vi "secuenciabloqueante.vi"() -> ()   [LabVIEW 2020]
panel:
  out "Boolean 2":bool
  in  "Boolean":bool
  out "Thermometer":dbl(slide) scale=0.0..100.0
  in  "stop":bool
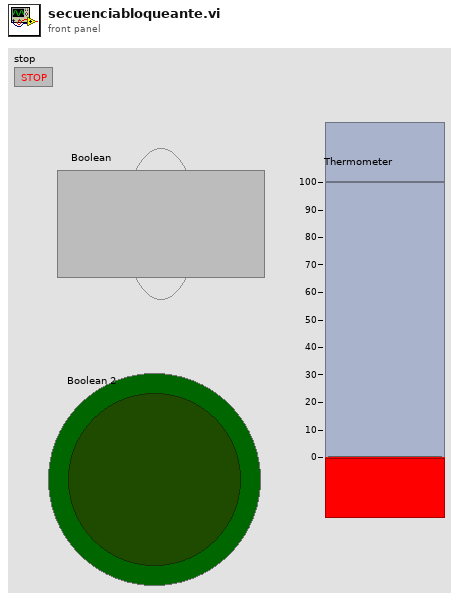
[diagram p1: front panel]
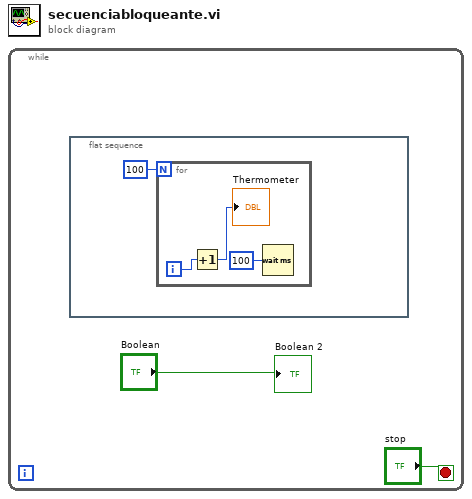
[diagram p0: block diagram]
diagram:
  n1 = while {
    stop <- "stop" stop-if-true
    n2 = flat-sequence {
      frame #0 {
        n3 = for {
          N: 100 -> [_]
          i -> [w6]
          n4 = Increment(x=w6) -> (x+1=→"Thermometer":i32)
          n5 = Wait (ms)(milliseconds to wait=u32 100) -> ()  [unwired: 1 out]
        }
      }
    }
    "Boolean 2" <- "Boolean"
  }
